vi "Event Msg To Nested.vi"(8 "Alias":string, 10 "Event":refnum<class "Event.lvclass">, 11 "Queue Actor in":refnum<class "Queue Actor.lvclass">) -> (0 "error out":errorcluster)   [LabVIEW 2021, in "Queue Actor.lvclass"]
uses:
  Queue Actor.lvclass
  Event/Event.lvclass
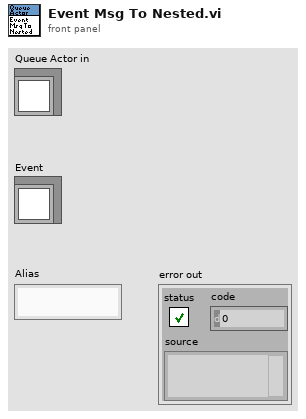
[diagram p1: front panel]
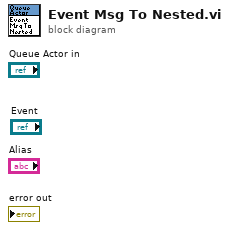
[diagram p0: block diagram]
diagram:
